vi "Open.vi"(8 "Error In":errorcluster, 11 "Keithley 7001 In":refnum<visa-resource-name>="GPIB0::7::INSTR") -> (0 "Error Out":errorcluster, 3 "Keithley 7001 Out":refnum<visa-resource-name>)   [LabVIEW 2012, in "Keithley-7001.lvlib"]
uses:
  Keithley-7001.lvlib
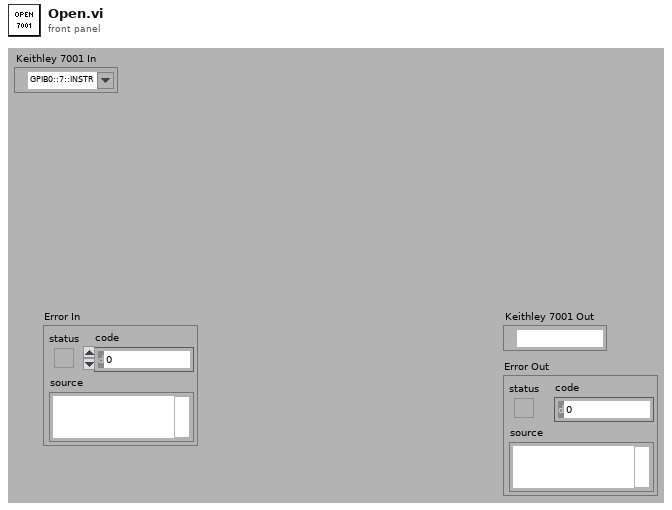
[diagram p1: front panel]
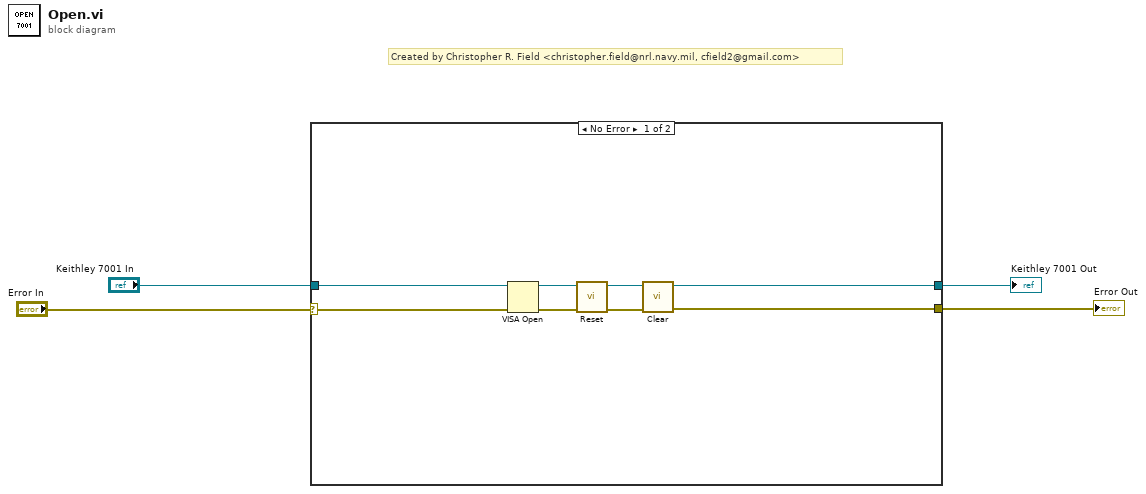
[diagram p0: block diagram]
diagram:
  # "Created by Christopher R. Field <christopher.field@nrl.navy.mil, cfield2@gmail.com>"
  n1 = case shown="No Error" "Error In" {
    selector: "Error In" -> [w5 w13]
    tunnel: "Keithley 7001 In" -> [w12 w14]
    tunnel: [w7 w14] -> w3
    tunnel: [w6 w13] -> w2
    frame No Error {
      n2 = VISA Open(error in (no error)=w5, VISA resource name=w12) -> (VISA resource name=w11:refnum<visa-resource-name>, error out=w10:errorcluster)  [unwired: 3 in]
      n3 = call "Reset.vi"("Error In"=w10, "Keithley 7001 In"=w11) -> ("Error Out"=w8:errorcluster, "Keithley 7001 Out"=w9:refnum<visa-resource-name>)  [unwired: 8 in]
      n4 = call "Clear.vi"("Error In"=w8, "Keithley 7001 In"=w9) -> ("Error Out"=w6:errorcluster, "Keithley 7001 Out"=w7:refnum<visa-resource-name>)  [unwired: 8 in]
    }
    frame Error {
    }
  }
  "Keithley 7001 Out" <- w3
  "Error Out" <- w2
